vi "UI Event-Settings-Value Change.vi"(8 "Error In":errorcluster, 11 "Root Panel Actor in":refnum<class "Root Panel Actor.lvclass">) -> (0 "Error Out":errorcluster, 3 "Root Panel Actor out":refnum<class "Root Panel Actor.lvclass">)   [LabVIEW 2021, in "Root Panel.lvlib" / "Root Panel Actor.lvclass"]
uses:
  Root Panel Actor.lvclass
  C:/Program Files (x86)/National Instruments/LabVIEW 2021/vi.lib/MGI/Panel Manager/Panel Actor/Panel Actor/Panel Actor.lvclass
  C:/Users/Thomas/Documents/Projects/TemplateVIEW/Sources/Appearance Actor/Appearance Actor/Appearance Actor.lvclass
  Modules/Settings Module/Settings Actor/Settings Actor.lvclass
  Root Panel Actor.lvclass/Root Panel Actor.ctl
  Appearance Actor/Appearance Actor/Appearance Actor.lvclass/Appearance Actor.ctl
  Appearance Actor/Appearance Actor Messages/Recieve Theme From Caller Msg/Recieve Theme From Caller Msg.lvclass/Recieve Theme From Caller Msg.ctl
  <vilib>/ActorFramework/Message Enqueuer/Message Enqueuer.lvclass/Message Enqueuer.ctl
  <vilib>/ActorFramework/Message Enqueuer/Enqueue.vi
  <vilib>/MGI/Panel Manager/Panel/Panel/Subpanel/Subpanel.lvclass
  C:/Program Files (x86)/National Instruments/LabVIEW 2021/vi.lib/MGI/Panel Manager/Panel/Panel/Panel.lvclass
  Appearance Actor/Appearance Actor Messages/Recieve Theme From Caller Msg/Recieve Theme From Caller Msg.lvclass
  C:/Program Files (x86)/National Instruments/LabVIEW 2021/vi.lib/ActorFramework/Message/Message.lvclass
  <vilib>/MGI/Panel Manager/Panel/Panel/Subpanel/Subpanel.vi
  <vilib>/ActorFramework/Message Priority Queue/Priority Enqueue.vi
  Appearance Actor/Theme Classes/Generic Theme/Generic Theme.lvclass
  <vilib>/MGI/Panel Manager/Panel Actor/Panel Actor/Panel Actor.lvclass
  <vilib>/MGI/Panel Manager/Panel/Panel.lvlib
  Appearance Actor/Appearance Actor/Appearance Actor.lvclass
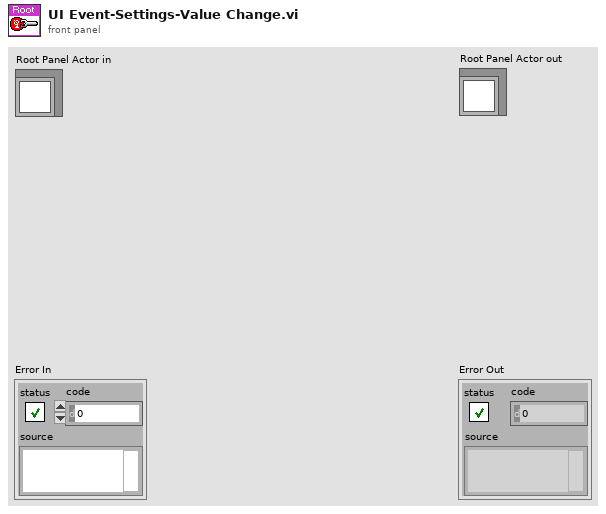
[diagram p1: front panel]
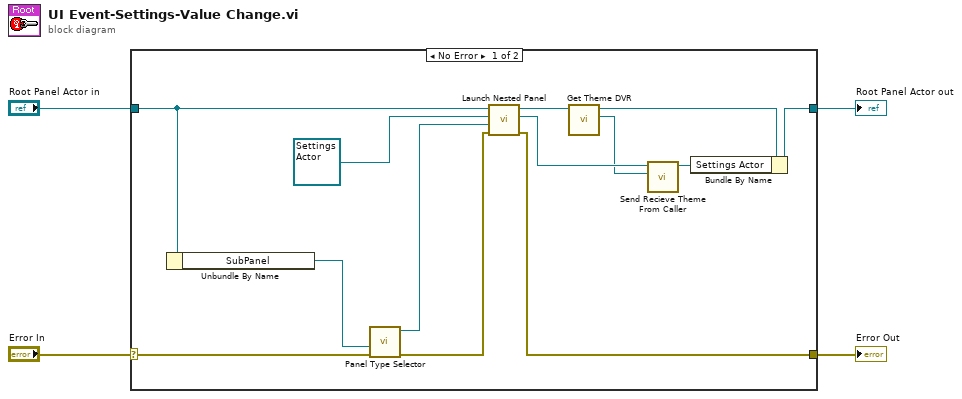
[diagram p0: block diagram]
diagram:
  n1 = case shown="No Error" "Error In" {
    selector: "Error In" -> [w15 w19]
    tunnel: [w16 w19] -> w1
    tunnel: [w17 w18] -> w3
    tunnel: "Root Panel Actor in" -> [w11 w18]
    frame No Error {
      n2 = Unbundle By Name(w11) -> ("SubPanel"=w10:refnum<vi>)
      n3 = call-poly <vilib>:"Panel Type Selector.vi"("Error In"=w15, "Sub Panel"=w10) -> ("Error Out"=w14:errorcluster, "Subpanel Out"=w13:refnum<class "Subpanel.lvclass">)  [unwired: 8 in]
      n4 = call <vilib>:"Launch Nested Panel.vi"("error in (no error)"=w14, "Panel"=w13, "Nested Panel Actor"=refnum<class "Settings Actor.lvclass"> refnum ("Settings Module.lvlib:Settings Actor.lvclass"), "Panel Actor in"=w11) -> ("error out"=w16:errorcluster, "Nested Actor's Enqueuer"=w9:refnum<class "Message Enqueuer.lvclass">, "Panel Actor out"=w7:refnum<class "Root Panel Actor.lvclass">)  [unwired: 4 in, 1 out]
      n5 = call "Get Theme DVR.vi"("Appearance Actor in"=w7) -> ("Theme DVR"=w5:refnum<data-value>, "Appearance Actor out"=w6:refnum<class "Root Panel Actor.lvclass">)  [unwired: 8 in, 1 out]
      n6 = call "Send Recieve Theme From Caller.vi"("Theme DVR"=w5, "Message Enqueuer"=w9) -> ("Message Enqueuer out"=w8:refnum<class "Message Enqueuer.lvclass">)  [unwired: 8 in, 1 out]
      n7 = Bundle By Name(cluster=w6, "Settings Actor"=w8) -> (w17:refnum<class "Root Panel Actor.lvclass">)
    }
    frame Error {
    }
  }
  "Error Out" <- w1
  "Root Panel Actor out" <- w3
